vi "test--chessboard GUI objects.vi"() -> ()   [LabVIEW 2018, in "main.lvlib"]
uses:
  main.lvlib
panel:
  in  "Chessboard":bool[][](array[boolean])
  in  "Array 3":bool[][](array[boolean])
  out "Array 2":bool[][](array[boolean])
  out "LED":bool
  out "Array":bool[][](array[boolean])
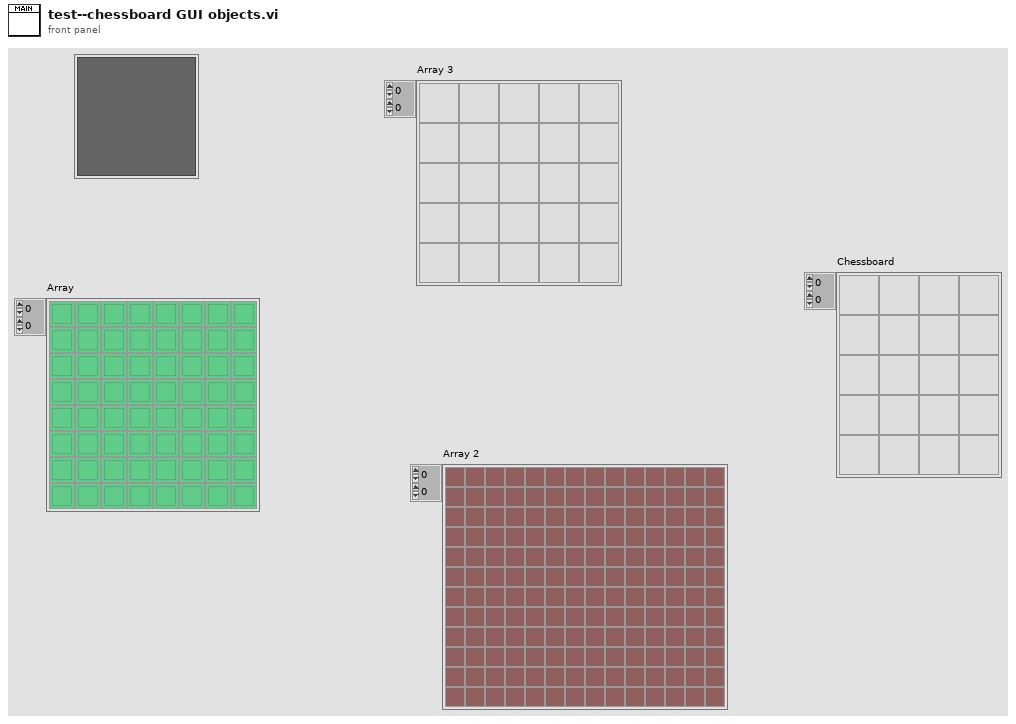
[diagram p1: front panel]
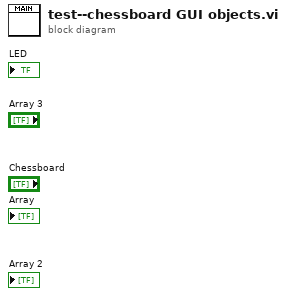
[diagram p0: block diagram]
diagram:
